vi "MFLI frontend V2.vi"(5 "Address":string="DEV3523", 13 "delay (msec)":i64=2) -> ()   [LabVIEW 2017]
uses:
  MFLI frontend action.ctl
  MFLI controller action.ctl
  publisher action.ctl
  Q - not nan -- real.vi
  <instrlib>/Zurich Instruments LabOne/Zurich Instruments LabOne.lvlib
panel:
  in  "save data":enum32{"main"}(tab)
  out "Selected Device":string="DEV3523"
  out "z out (V)":cdb
  out "Freq out (Hz)":dbl
  in  "MFLI frontend action":T1
  in  "stop!":bool
  out "Selected Device 2":string="DEV3523"
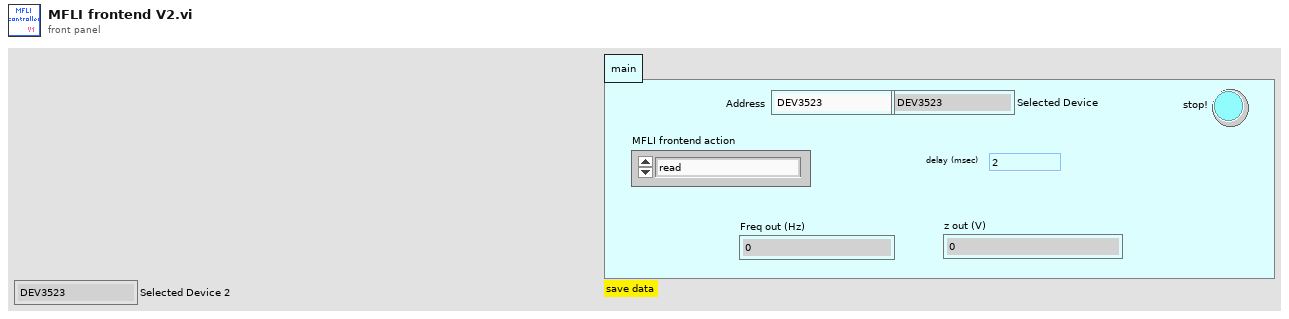
[diagram p1: front panel]
types:
  T1 = typedef "MFLI frontend action.ctl" = enum16{"read", "writeread", "open", "close"}
  T2 = typedef "MFLI controller action.ctl" = enum16{"Initialize", "Scan frequency", "open", "close", "read", "circle PLL"}
  T3 = typedef "Zurich Instruments LabOne.lvlib/ziTypeHandle.ctl" = cluster{"handleValid":bool, "Conn":u64, "Path Prefix":string, "Handle":u64, "Connected":bool, "Clockbase(s)":dbl}
  T4 = typedef "publisher action.ctl" = enum16{"set", "get"}
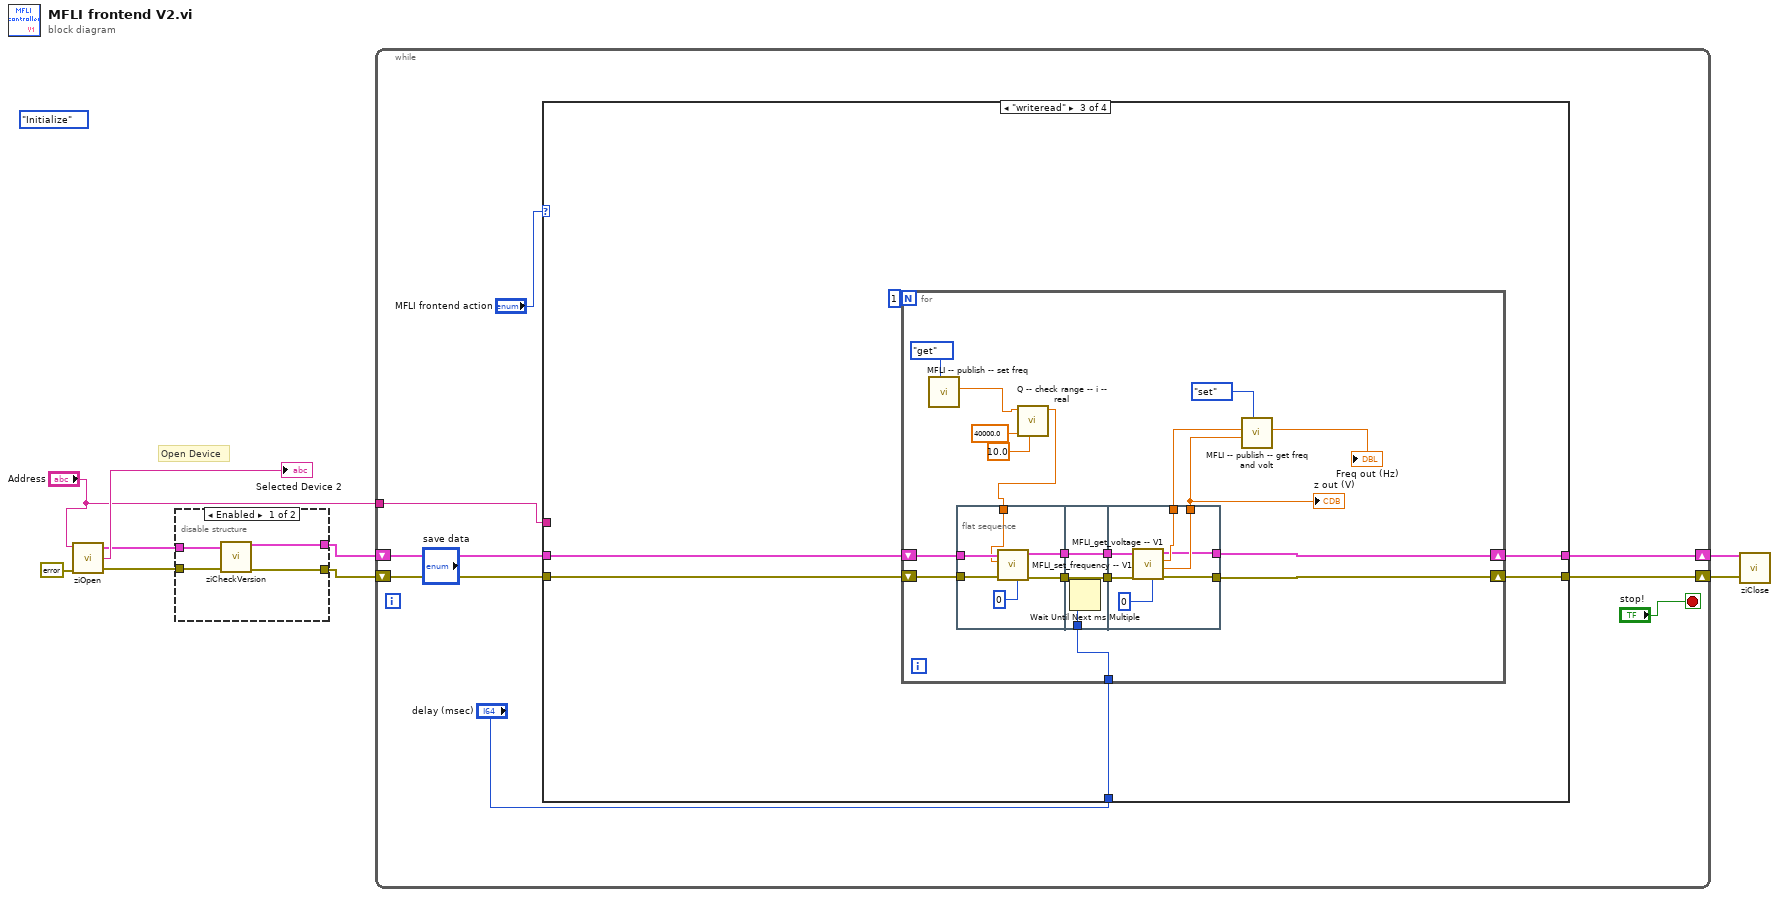
[diagram p0: block diagram]
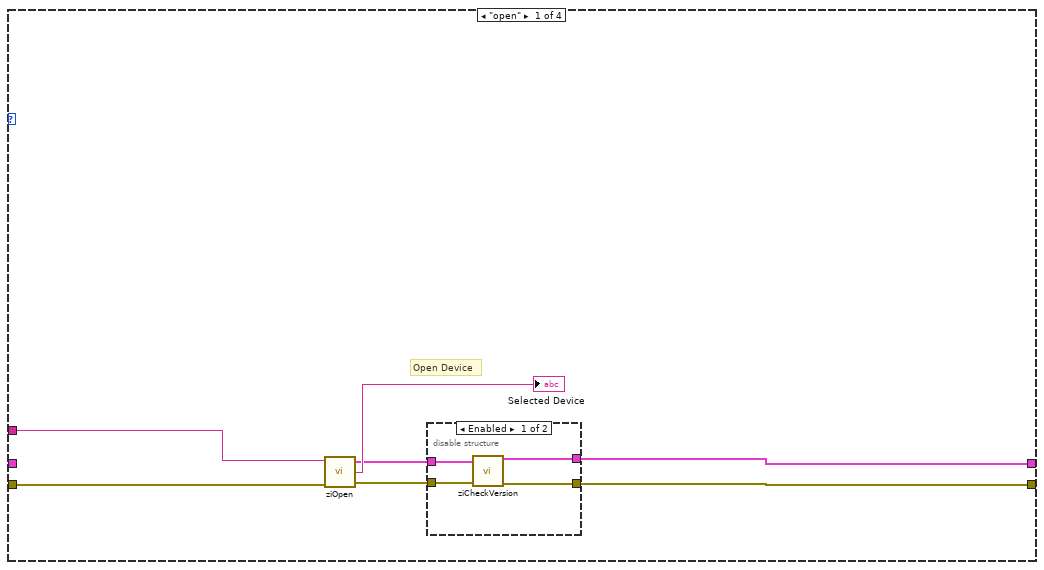
[diagram p3: hidden frame]
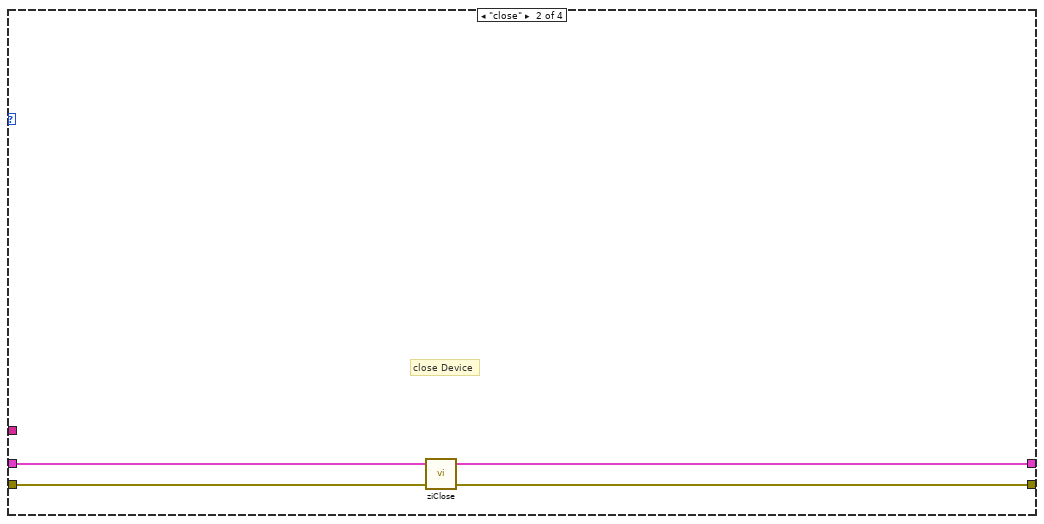
[diagram p5: hidden frame]
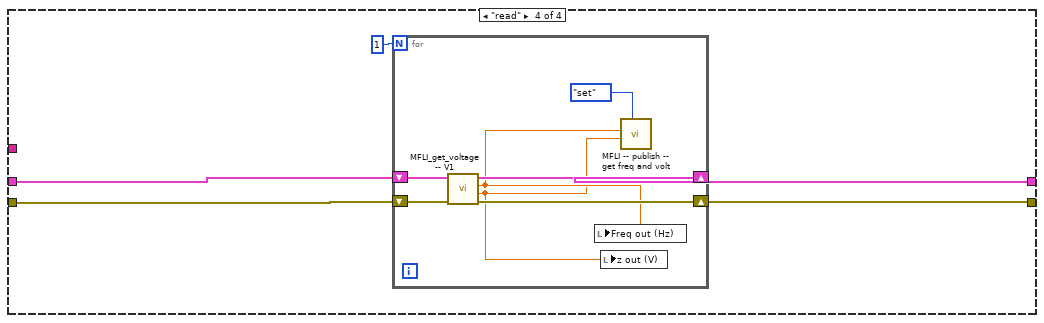
[diagram p6: hidden frame]
diagram:
  (unwired) MFLI_controller_action."Initialize" ("MFLI controller action")
  # "Open Device"
  n1 = call <instrlib>:"ziOpen.vi"("Error In"=errorcluster {"status"=FALSE, "code"=0, "source"=""}, "Address"="Address") -> ("Error Out"=w9:errorcluster, "Selected Device"=→"Selected Device 2":string, "HandleOut"=w7:T3)  [unwired: 2 in]
  n2 = disable-structure shown="Enabled" {
    disable-tunnel: w9 -> [w13 w14]
    disable-tunnel: [w12 w14] -> w3
    disable-tunnel: [w11 w15] -> w4
    disable-tunnel: w7 -> [w10 w15]
    frame Enabled {
      n3 = call <instrlib>:"ziCheckVersion.vi"("Handle In"=w10, "Error In"=w13) -> ("Handle Out"=w11:T3, "Error Out"=w12:errorcluster)  [unwired: 12 in]
    }
    frame Disabled {
    }
  }
  n4 = while {
    shift-right: [w22] -> w2
    shift-left: w4 -> [w23]
    shift-right: [w21] -> w1
    shift-left: w3 -> [w20]
    tunnel: "Address" -> [w17]
    stop <- "stop!" stop-if-true
    n5 = case shown="\"writeread\"" "MFLI frontend action" {
      tunnel: w23 -> [_ w39 w46 w84]
      tunnel: w20 -> [w27 w40 w45 w83]
      tunnel: w17 -> [w28 _ _ _]
      tunnel: "delay (msec)" -> [_ _ w44 _]
      tunnel: [w25 w38 w42 w80] -> w22
      tunnel: [w24 w37 w41 w81] -> w21
      frame "open" {
        # "Open Device"
        n6 = call <instrlib>:"ziOpen.vi"("Error In"=w27, "Address"=w28) -> ("Error Out"=w30:errorcluster, "Selected Device"=→"Selected Device":string, "HandleOut"=w26:T3)  [unwired: 2 in]
        n7 = disable-structure shown="Enabled" {
          disable-tunnel: w30 -> [w34 w35]
          disable-tunnel: [w33 w35] -> w24
          disable-tunnel: [w32 w36] -> w25
          disable-tunnel: w26 -> [w31 w36]
          frame Enabled {
            n8 = call <instrlib>:"ziCheckVersion.vi"("Handle In"=w31, "Error In"=w34) -> ("Handle Out"=w32:T3, "Error Out"=w33:errorcluster)  [unwired: 12 in]
          }
          frame Disabled {
          }
        }
      }
      frame "close" {
        # "close Device"
        n9 = call <instrlib>:"ziClose.vi"("Error In"=w40, "Handle In"=w39) -> ("Error Out"=w37:errorcluster, "Handle Out"=w38:T3)  [unwired: 2 in]
      }
      frame "writeread" {
        n10 = for {
          N: 1 -> [_]
          shift-right: [w56] -> w42
          shift-left: w46 -> [w63]
          shift-right: [w55] -> w41
          shift-left: w45 -> [w62]
          tunnel: w44 -> [w57]
          n11 = call "MFLI -- publish -- set freq.vi"("publisher action"=publisher_action."get") -> ("freq out (Hz)"=w50:dbl)  [unwired: 10 in]
          n12 = flat-sequence {
            tunnel: w63 -> [w69]
            tunnel: w62 -> [w67]
            tunnel: [w68] -> w61
            tunnel: [w66] -> w60
            tunnel: w47 -> [w64]
            tunnel: w61 -> [w71]
            tunnel: w60 -> [w72]
            tunnel: [w71] -> w59
            tunnel: [w72] -> w58
            tunnel: w57 -> [w70]
            tunnel: [w73] -> w55
            tunnel: w59 -> [w76]
            tunnel: w58 -> [w74]
            tunnel: [w79] -> w52
            tunnel: [w78] -> w51
            tunnel: [w75] -> w56
            frame #0 {
              n13 = call "MFLI_set_frequency -- V1.vi"("Oscillator (0)"=u16 0, "Error In"=w67, "Freq in (Hz)"=w64, "Handle In"=w69) -> ("Error Out"=w66:errorcluster, "Handle Out"=w68:T3)  [unwired: 4 in, 2 out]
            }
            frame #1 {
              n14 = Wait Until Next ms Multiple(millisecond multiple=w70) -> ()  [unwired: 1 out]
            }
            frame #2 {
              n15 = call "MFLI_get_voltage -- V1.vi"("Oscillator (0)"=u16 0, "Error In"=w74, "Handle In"=w76) -> ("Error Out"=w73:errorcluster, "z out (V)"=w78:cdb, "Freq out (Hz)"=w79:dbl, "Handle Out"=w75:T3)  [unwired: 5 in]
            }
          }
          n16 = call "Q -- check range -- i -- real.vi"("lower"=10.0, "default"=40000.0, "number"=w50) -> ("number in range"=w47:dbl)  [unwired: 6 in, 2 out]
          n17 = call "MFLI -- publish -- get freq and volt.vi"("publisher action"=publisher_action."set", "Voltage IN (V)"=w51, "freq IN (Hz)"=w52) -> ()  [unwired: 7 in, 2 out]
          "z out (V)" <- w51
          "Freq out (Hz)" <- w52
        }
      }
      frame "read" {
        n18 = for {
          N: 1 -> [_]
          shift-right: [w90] -> w81
          shift-left: w83 -> [w91]
          shift-right: [w88] -> w80
          shift-left: w84 -> [w89]
          n19 = call "MFLI_get_voltage -- V1.vi"("Error In"=w91, "Handle In"=w89) -> ("Error Out"=w90:errorcluster, "z out (V)"=w85:cdb, "Freq out (Hz)"=w86:dbl, "Handle Out"=w88:T3)  [unwired: 6 in]
          n20 = local write "Freq out (Hz)"(w86) -> ()
          n21 = local write "z out (V)"(w85) -> ()
          n22 = call "MFLI -- publish -- get freq and volt.vi"("publisher action"=publisher_action."set", "Voltage IN (V)"=w85, "freq IN (Hz)"=w86) -> ()  [unwired: 7 in, 2 out]
        }
      }
    }
  }
  n23 = call <instrlib>:"ziClose.vi"("Error In"=w1, "Handle In"=w2) -> ()  [unwired: 2 in, 2 out]
